vi "Write then read.vi"(7 "Max bytes to read (999)":u32=999, 8 "error in (no error)":errorcluster, 9 "Trim RX? (T)":bool, 10 "TX Data":string, 11 "Serial Device in":refnum<class "Serial Device.lvclass">) -> (0 "error out":errorcluster, 2 "RX Data":string, 3 "Serial Device out":refnum<class "Serial Device.lvclass">)   [LabVIEW 2015, in "Serial Device.lvclass"]
uses:
  Serial Device.lvclass
  Serial Device.lvclass/Serial Device.ctl
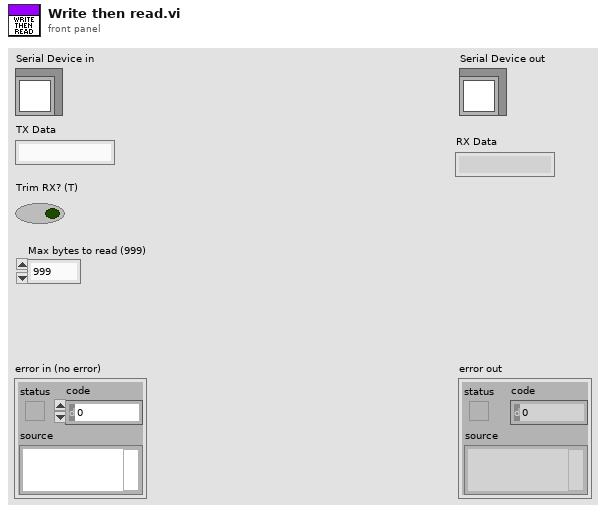
[diagram p1: front panel]
types:
  T1 = typedef "Semaphore RefNum" = refnum<k1>
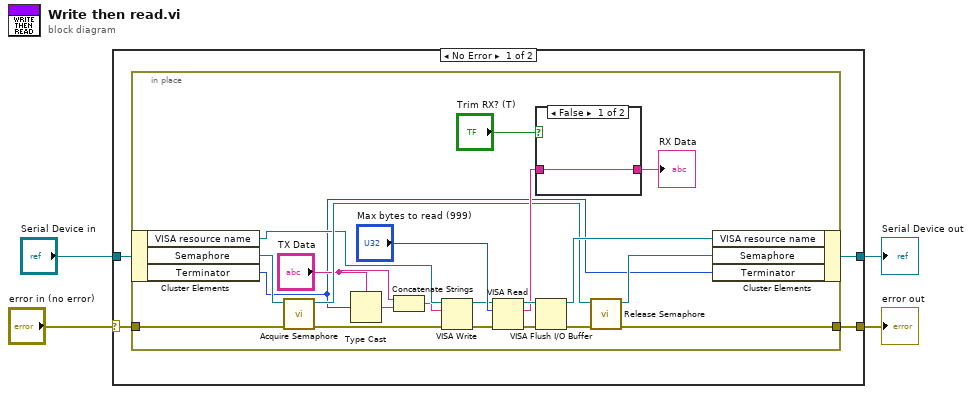
[diagram p0: block diagram]
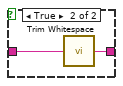
[diagram p2: hidden frame]
diagram:
  n1 = case shown="No Error" "error in (no error)" {
    selector: "error in (no error)" -> [w8 w34]
    tunnel: [w5 w34] -> w3
    tunnel: [w6 w33] -> w1
    tunnel: "Serial Device in" -> [w7 w33]
    frame No Error {
      n2 = in-place {
        in-place-border: w8 -> [w28]
        in-place-border: [w18] -> w5
        n3 = in-place-cluster #1(w7) -> ("VISA resource name"=w13:refnum<visa-resource-name>, "Semaphore"=w27:T1, "Terminator"=w9:u8)
        n4 = call <vilib>:"Acquire Semaphore.vi"("error in (no error)"=w28, "semaphore"=w27) -> ("error out"=w16:errorcluster, "semaphore out"=w19:T1)  [unwired: 3 in, 1 out]
        n5 = Type Cast(type="TX Data", x=w9) -> (*(type *) &x=w10:string)
        n6 = Concatenate Strings("TX Data", w10) -> (w12:string)
        n7 = VISA Write(VISA resource name=w13, write buffer=w12, error in (no error)=w16) -> (VISA resource name out=w14:refnum<visa-resource-name>, error out=w15:errorcluster)  [unwired: 1 out]
        n8 = VISA Read(VISA resource name=w14, byte count="Max bytes to read (999)", error in (no error)=w15) -> (VISA resource name out=w26:refnum<visa-resource-name>, read buffer=w23:string, error out=w21:errorcluster)  [unwired: 1 out]
        n9 = case shown="False" "Trim RX? (T)" {
          tunnel: [w30 w32] -> w24
          tunnel: w23 -> [w30 w31]
          frame False {
          }
          frame True {
            n10 = call <vilib>:"Trim Whitespace.vi"("string"=w31) -> ("trimmed string"=w32:string)  [unwired: 1 in]
          }
        }
        "RX Data" <- w24
        n11 = VISA Flush I/O Buffer(VISA resource name=w26, error in (no error)=w21) -> (VISA resource name out=w25:refnum<visa-resource-name>, error out=w22:errorcluster)  [unwired: 1 in]
        n12 = call <vilib>:"Release Semaphore.vi"("error in (no error)"=w22, "semaphore"=w19) -> ("error out"=w18:errorcluster, "semaphore out"=w20:T1)  [unwired: 4 in]
        n13 = in-place-cluster #1("VISA resource name"=w25, "Semaphore"=w20, "Terminator"=w9) -> (w6:refnum<class "Serial Device.lvclass">)
      }
    }
    frame Error {
    }
  }
  "error out" <- w3
  "Serial Device out" <- w1
